vi "WAV CFG.vi"(0 "System no.":i32=1 min=1 max=4 step=1, 2 "Affected axes":string[](array[string]), 3 "WAV CFG parameters":T1={"n"=1000, "m"=1, "p"=0, "k"=0, "s"=0.0, "L"=0.0} {"L" format="%.6f"; "s" format="%.6f"}, 4 "No.of digits\nfor s and L":i16=3, 5 "error in":errorcluster) -> (14 "Controller error":bool, 19 "error out":errorcluster)   [LabVIEW 2026]
doc: "This VI configures a wave generator for one or more axes. Controller error is TRUE if selected system reports an error code which is not zero. Please refer to the system manual for a description of wave generator configuration parameters, units and restrictions.\n\nE-516, E-761: Only one axis per command allowed.\n\nE-517, E-518: Affected axis is identical with wave table number, which can be 1 to 3. Only one wave table per command allowed."
uses:
  GeneralCommands/Controller names.ctl
  GeneralCommands/Global2 (Array).vi
panel:
  # "This vi configures a wave generator for one or more axes. Please\nrefer to the system manual for a description of wave generator\nconfiguration parameters, units and restrictions."
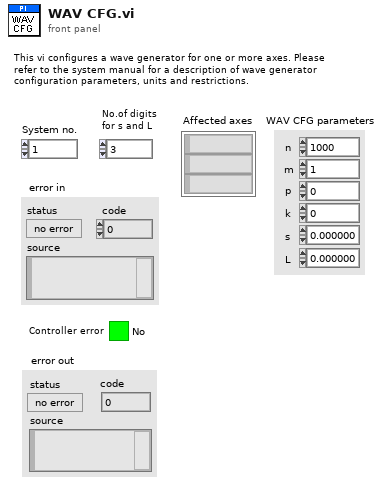
[diagram p1: front panel]
types:
  T1 = cluster{"n":i32, "m":i32, "p":i32, "k":i32, "s":dbl, "L":dbl}
  T2 = typedef "Controller names.ctl" = enum16{"None", "Analog", "C-702", "C-413", "C-414", "C-843", "C-843.PM", "C-844", "C-848", "C-865", "C-866", "C-867", "C-877", "C-880", "C-884", "C-885", "C-886", "C-887", "C-891", "E-135", "E-516", "E-517", "E-518", "E-709", "E-710", "E-712", "E-725", "E-727", "E-753", "E-754", "E-755", "E-761", "E-816", "E-861", "E-870", "E-871", "E-872", "E-873", "E-874", "F-206", "HydraPollux", "M-840", "M-850", "M-8X0", "Mercury", "Mercury_GCS", "PI_GCS2"}
  T3 = cluster{"Conn. axes":string[], "Controller name":T2}[]
  T4 = cluster{"Conn. axes":string[], "Controller name":T2}
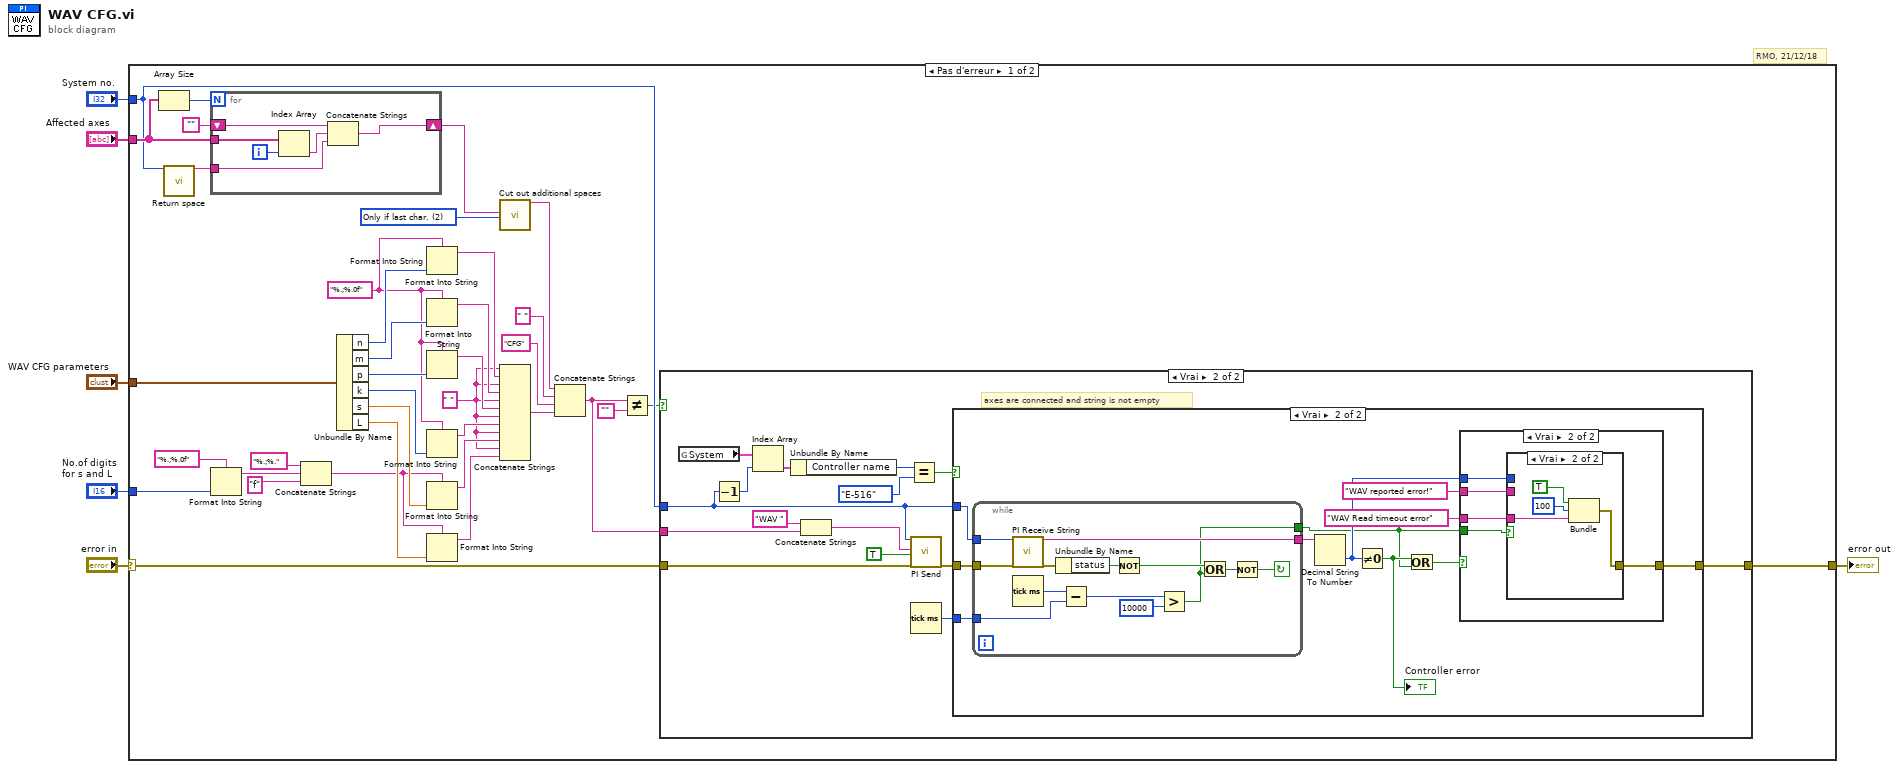
[diagram p0: block diagram]
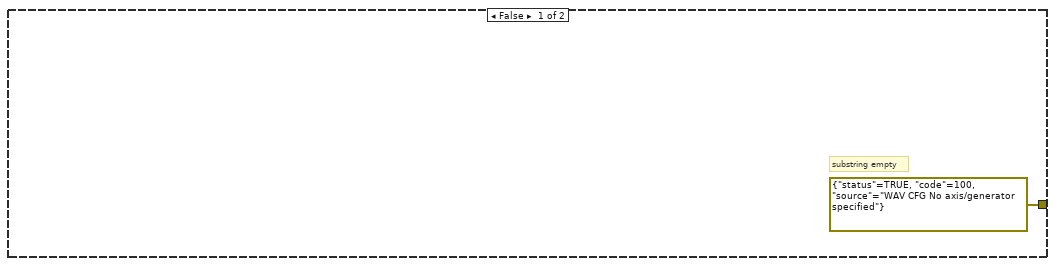
[diagram p2: hidden frame]
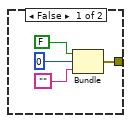
[diagram p4: hidden frame]
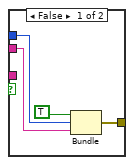
[diagram p5: hidden frame]
diagram:
  # "RMO, 21/12/18"
  n1 = case shown="Pas d'erreur" "error in" {
    selector: "error in" -> [w7 w108]
    tunnel: [w43 w108] -> w6
    tunnel: "System no." -> [w19 _]
    tunnel: "Affected axes" -> [w39 _]
    tunnel: "WAV CFG parameters" -> [w26 _]
    tunnel: "No.of digits\nfor s and L" -> [w10 _]
    frame No Error {
      w17 = u16 2 items=["All Spaces", "Only if 1st char.", "Only if last char.", "Only if near \"=\"", "Only if 1st or last char.", "Only multiple"] ("Mode")
      w25 = "%.;%.0f" ("Format String")
      w24 = " " ("Substring")
      n2 = Array Size(array=w39) -> (size(s)=w41:i32)
      n3 = call "Return space.vi"("System no."=w19) -> ("String out"=w18:string)  [unwired: 1 in, 17 out]
      n4 = for {
        N: w41 -> [_]
        tunnel: w39 -> [w48]
        shift-right: [w47] -> w16
        shift-left: "" -> [w45]
        tunnel: w18 -> [w44]
        i -> [w49]
        n5 = Index Array(array=w48, index=w49) -> (element=w46:string)
        n6 = Concatenate Strings(w45, w46, w44) -> (w47:string)
      }
      n7 = Format Into String(format string="%.;%.0f" ("Format String"), w10) -> (resulting string=w11:string)  [unwired: 2 in, 1 out]
      n8 = Concatenate Strings("%.;%." ("Format String"), w11, "f" ("Format String")) -> (w9:string)
      n9 = Unbundle By Name(w26) -> ("n"=w38:i32, "m"=w37:i32, "p"=w36:i32, "k"=w35:i32, "s"=w34:dbl, "L"=w28:dbl)
      n10 = Format Into String(format string=w25, w38) -> (resulting string=w33:string)  [unwired: 2 in, 1 out]
      n11 = Format Into String(format string=w25, w37) -> (resulting string=w32:string)  [unwired: 2 in, 1 out]
      n12 = Format Into String(format string=w25, w36) -> (resulting string=w31:string)  [unwired: 2 in, 1 out]
      n13 = Format Into String(format string=w25, w35) -> (resulting string=w30:string)  [unwired: 2 in, 1 out]
      n14 = Format Into String(format string=w9, w34) -> (resulting string=w29:string)  [unwired: 2 in, 1 out]
      n15 = Format Into String(format string=w9, w28) -> (resulting string=w27:string)  [unwired: 2 in, 1 out]
      n16 = call "Cut out additional spaces.vi"("String"=w16, "Mode"=w17) -> ("String out"=w15:string)  [unwired: 17 out]
      n17 = Concatenate Strings(w24, w33, w24, w32, w24, w31, w24, w30, w24, w29, w24, w27) -> (w22:string)
      n18 = Concatenate Strings(w15, " " ("Substring"), "CFG", w22) -> (w23:string)
      n19 = Not Equal?(x=w23, y="") -> (x != y?=w8:bool)
      n20 = case shown="Vrai" w8 {
        tunnel: w23 -> [_ w64]
        tunnel: [errorcluster {"status"=TRUE, "code"=100, "source"="WAV CFG No axis/generator specified"} ("error out") w58] -> w43
        tunnel: w7 -> [_ w61]
        tunnel: w19 -> [_ w52]
        frame False {
          # "substring empty"
        }
        frame True {
          # "axes are connected and string is not empty"
          n21 = global read "Global2 (Array).vi" "System"() -> (w56:T3)
          n22 = Decrement(x=w52) -> (x-1=w55:i32)
          n23 = Index Array(array=w56, index=w55) -> (element=w54:T4)
          n24 = Unbundle By Name(w54) -> ("Controller name"=w53:T2)
          n25 = Concatenate Strings("WAV ", w64) -> (w62:string)
          n26 = Equal?(x=w53, y=Controller_names."E-516" ("System 1")) -> (x = y?=w51:bool)
          n27 = call "PI Send.vi"("System no."=w52, "String to send"=w62, "Attach termination char.?"=TRUE ("Attach Linefeed?"), "error in"=w61) -> ("error out"=w59:errorcluster)  [unwired: 2 in, 13 out]
          n28 = Tick Count (ms)() -> (millisecond timer value=w60:u32)
          n29 = case shown="Vrai" w51 {
            tunnel: w60 -> [_ w77]
            tunnel: w59 -> [w66 w76]
            tunnel: w52 -> [_ w75]
            tunnel: [w66 w70] -> w58
            frame False {
            }
            frame True {
              n30 = while {
                tunnel: [w78] -> w68
                tunnel: [w79] -> w74
                tunnel: w75 -> [w80]
                tunnel: w76 -> [w81]
                tunnel: w77 -> [w82]
                stop <- w83 continue-if-true
                n31 = call "PI Receive String.vi"("System no."=w80, "error in"=w81) -> ("String read"=w79:string, "error out"=w90:errorcluster)  [unwired: 1 in, 15 out]
                n32 = Tick Count (ms)() -> (millisecond timer value=w88:u32)
                n33 = Unbundle By Name(w90) -> ("status"=w89:bool)
                n34 = Subtract(x=w88, y=w82) -> (x-y=w87:u32)
                n35 = Not(x=w89) -> (.not. x?=w85:bool)
                n36 = Greater?(x=w87, y=u32 10000) -> (0:w78:bool)
                n37 = Or(x=w85, y=w78) -> (x .or. y?=w84:bool)
                n38 = Not(x=w84) -> (.not. x?=w83:bool)
              }
              n39 = Decimal String To Number(string=w74) -> (number=w72:i32)  [unwired: 3 out]
              n40 = Not Equal To 0?(x=w72) -> (x != 0?=w69:bool)
              "Controller error" <- w69
              n41 = Or(x=w69, y=w68) -> (x .or. y?=w67:bool)
              n42 = case shown="Vrai" w67 {
                tunnel: w68 -> [_ w99]
                tunnel: "WAV Read timeout error" -> [_ w98]
                tunnel: w72 -> [_ w97]
                tunnel: "WAV reported error!" -> [_ w96]
                tunnel: [w91 w95] -> w70
                frame False {
                  n43 = Bundle(FALSE, 0, "") -> (w91:errorcluster)  [unwired: 1 out]
                }
                frame True {
                  n44 = case shown="Vrai" w99 {
                    tunnel: w98 -> [_ w105]
                    tunnel: w97 -> [w102 _]
                    tunnel: w96 -> [w101 _]
                    tunnel: [w100 w104] -> w95
                    frame False {
                      n45 = Bundle(TRUE, w102, w101) -> (w100:errorcluster)  [unwired: 1 out]
                    }
                    frame True {
                      n46 = Bundle(TRUE, 100, w105) -> (w104:errorcluster)  [unwired: 1 out]
                    }
                  }
                }
              }
            }
          }
        }
      }
    }
    frame Error {
    }
  }
  "error out" <- w6
